vi "Pre Launch Init.vi"(11 "UDP_receiver in":refnum<class "UDP_receiver.lvclass">) -> (0 "error out":errorcluster, 3 "UDP_receiver out":refnum<class "UDP_receiver.lvclass">)   [LabVIEW 2025, in "UDP_receiver.lvlib" / "UDP_receiver.lvclass"]
doc: "(<B>Filename</B>: Actor Framework.lvlib:Actor.lvclass:Pre Launch Init.vi)\n\nDefines behavior that occurs after the Launch Nested Actor method is invoked but before the actor's Actor Core method begins running.\n\nBy default, this method does nothing. A descendant class may override it to define behavior."
uses:
  UDP_receiver.lvclass
  UDP_receiver.lvclass/UDP_receiver.ctl
  <vilib>/ActorFramework/Actor/Actor.lvclass
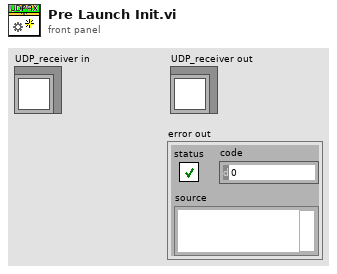
[diagram p1: front panel]
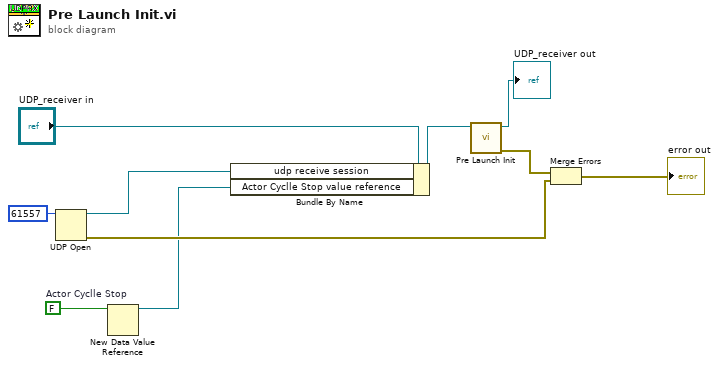
[diagram p0: block diagram]
diagram:
  w2 = FALSE  # Actor Cyclle Stop
  n1 = UDP Open(11:u16 61557 ("port")) -> (port=w7:refnum<k16>, 0:w4:errorcluster)  [unwired: 4 in, 1 out]
  n2 = New Data Value Reference(data value=w2) -> (data value reference=w1:refnum<data-value>)  [unwired: 1 in, 1 out]
  n3 = Bundle By Name(cluster="UDP_receiver in", "udp receive session"=w7, "Actor Cyclle Stop value reference"=w1) -> (w6:refnum<class "UDP_receiver.lvclass">)
  n4 = call-parent "Pre Launch Init.vi"("Actor in"=w6) -> ("error out"=w5:errorcluster, "Actor out"=→"UDP_receiver out":refnum<class "UDP_receiver.lvclass">)  [unwired: 9 in]
  n5 = Merge Errors(w5, w4) -> (→"error out":errorcluster)
